vi "Get Snapshot Block List.vi"(7 "Snapshot":string, 8 "error in (no error)":errorcluster, 9 "Blob":string, 10 "Container":string, 11 "Azure Session in":refnum<class "Session.lvclass">) -> (0 "error out":errorcluster, 1 "Uncommitted Blocks":string[](array[string]), 2 "Committed Blocks":string[](array[string]), 3 "Azure Session out":refnum<class "Session.lvclass">)   [LabVIEW 2015, in "NI_Azure_Blob.lvlib"]
doc: "Retrieves the list of blocks that have been uploaded as part of a snapshot of a block blob."
uses:
  NI_Azure_Blob.lvlib
  Core/Session/Session.lvclass
  Core/Name Value Pair.ctl
  Core/Session/Session.lvclass/Session.ctl
  Core/Session/Write HTTP Verb.vi
  Core/Session/Write URL Suffix.vi
  Core/Session/Write Request Parameters.vi
  Core/NI_Azure_Core.lvlib
  XML Parsing/NI_Azure_XML Parsing.lvlib
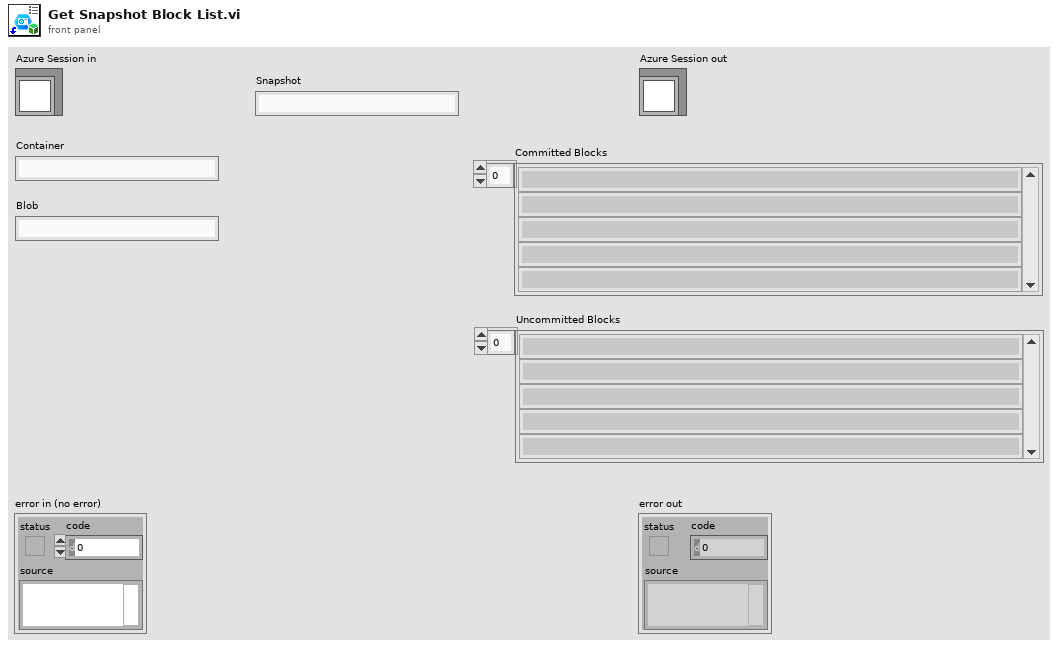
[diagram p1: front panel]
types:
  T1 = typedef "NI_Azure_Core.lvlib/Name Value Pair.ctl" = cluster{"name":string, "value":string}
  T2 = typedef "NI_Azure_Core.lvlib/Response.ctl" = cluster{"Headers":string, "Body":string}
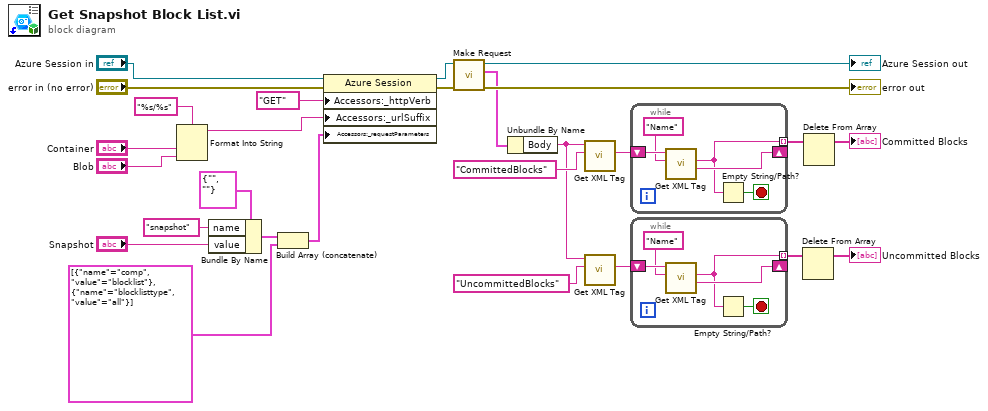
[diagram p0: block diagram]
diagram:
  n1 = Format Into String(format string="%s/%s", "Container", "Blob") -> (resulting string=w17:string)  [unwired: 2 in, 1 out]
  n2 = Bundle By Name(cluster=T1 {"name"="", "value"=""} ("Name Value Pair"), "name"="snapshot", "value"="Snapshot") -> (w4:T1)
  n3 = Build Array (concatenate)(w4, T1[] [{"name"="comp", "value"="blocklist"}, {"name"="blocklisttype", "value"="all"}] ("appended array")) -> (w1:T1[])
  n4 = property class="Azure Session"(reference="Azure Session in", error in="error in (no error)", "Accessors:_httpVerb"="GET" ("HTTP-Verb"), "Accessors:_urlSuffix"=w17, "Accessors:_requestParameters"=w1) -> (reference out=w21:refnum<class "Session.lvclass">, error out=w19:errorcluster)
  n5 = call "Make Request.vi"("error in (no error)"=w19, "Session in"=w21) -> ("error out"=→"error out":errorcluster, "Response"=w16:T2, "Session out"=→"Azure Session out":refnum<class "Session.lvclass">)  [unwired: 7 in]
  n6 = Unbundle By Name(w16) -> ("Body"=w11:string)
  n7 = call "Get XML Tag.vi"("Tag name"="CommittedBlocks", "XML String in"=w11) -> ("Tag value"=w15:string)  [unwired: 5 in, 4 out]
  n8 = call "Get XML Tag.vi"("Tag name"="UncommittedBlocks", "XML String in"=w11) -> ("Tag value"=w12:string)  [unwired: 5 in, 4 out]
  n9 = while {
    shift-right: [w31] -> _
    shift-left: w15 -> [w32]
    tunnel: [w29] -> w10 mode=indexing
    stop <- w28 stop-if-true
    n10 = call "Get XML Tag.vi"("Tag name"="Name", "XML String in"=w32) -> ("Remaining string"=w31:string, "Tag value"=w29:string)  [unwired: 5 in, 3 out]
    n11 = Empty String/Path?(string/path=w29) -> (empty?=w28:bool)
  }
  n12 = while {
    shift-right: [w36] -> _
    shift-left: w12 -> [w37]
    tunnel: [w34] -> w8 mode=indexing
    stop <- w33 stop-if-true
    n13 = call "Get XML Tag.vi"("Tag name"="Name", "XML String in"=w37) -> ("Remaining string"=w36:string, "Tag value"=w34:string)  [unwired: 5 in, 3 out]
    n14 = Empty String/Path?(string/path=w34) -> (empty?=w33:bool)
  }
  n15 = Delete From Array(array=w8) -> (array with subset deleted=→"Uncommitted Blocks":string[])  [unwired: 2 in, 1 out]
  n16 = Delete From Array(array=w10) -> (array with subset deleted=→"Committed Blocks":string[])  [unwired: 2 in, 1 out]
